vi "oa_TV Wait Until Ten Revs (NChan).vi"(5 "reset? (F)":bool, 8 "error in (no error)":errorcluster, 10 "pulse/revolution":i32[](array[numeric]), 11 "pulse position [s]":cluster{dbl[]}[](array[cluster]) {"?" format="%.2f"}) -> (0 "error out":errorcluster, 3 "pulse positions":cluster{dbl[]}[](array[cluster]))   [LabVIEW 2017, in "SoundVib_Torsional.lvlib"]
uses:
  <vilib>/addons/Sound and Vibration/Order Analysis/Torsional Vibration/SoundVib_Torsional.lvlib
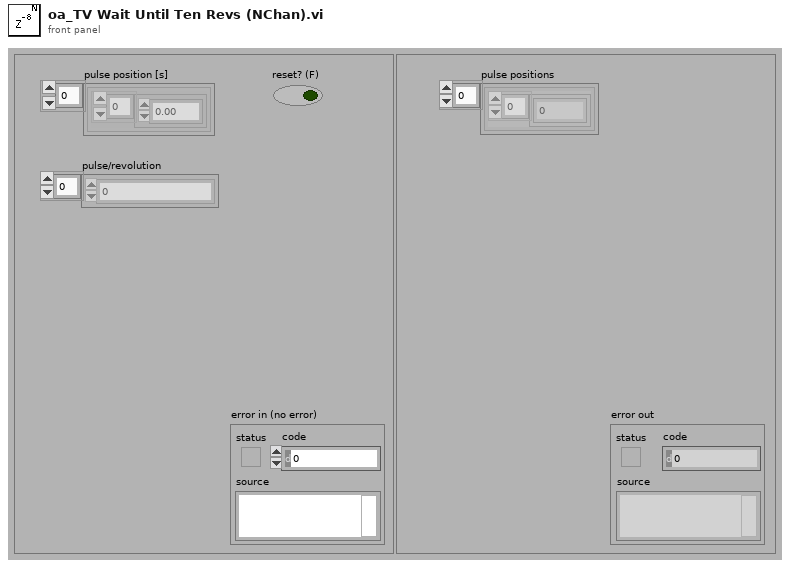
[diagram p1: front panel]
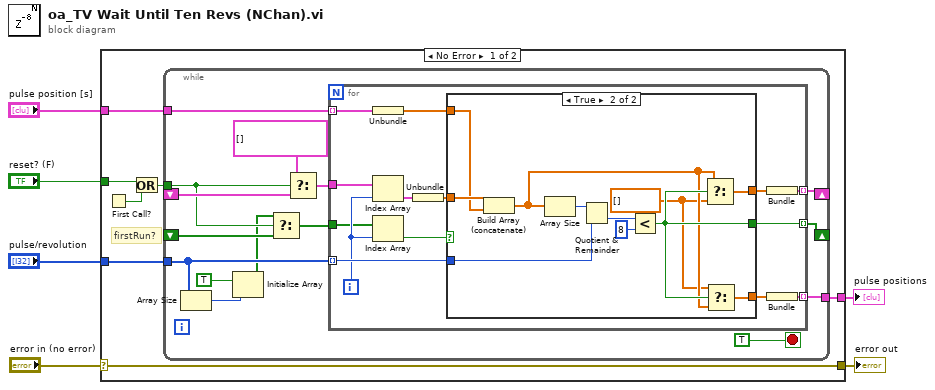
[diagram p0: block diagram]
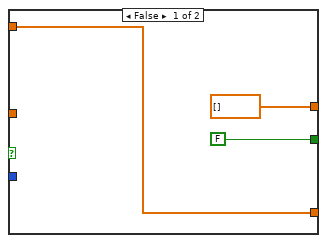
[diagram p2: hidden frame]
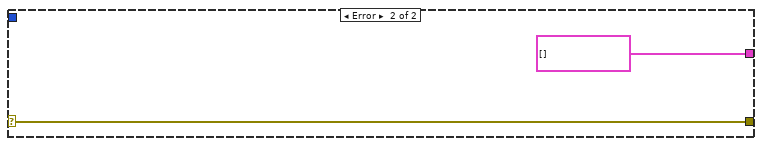
[diagram p3: hidden frame]
diagram:
  n1 = case shown="No Error" "error in (no error)" {
    selector: "error in (no error)" -> [w13 w58]
    tunnel: [w13 w58] -> w5
    tunnel: [w12 cluster{"f":dbl[]}[] []] -> w1
    tunnel: "reset? (F)" -> [w10 _]
    tunnel: "pulse position [s]" -> [w8 _]
    tunnel: "pulse/revolution" -> [w7 _]
    frame No Error {
      # "firstRun?"
      n2 = First Call?() -> (First Call?: T/F=w11:bool)
      n3 = Or(x=w10, y=w11) -> (x .or. y?=w9:bool)
      n4 = while {
        shift-right: [w24] -> _
        shift-left: _ -> [w23]
        tunnel: w9 -> [w19]
        shift-right: [w26] -> _
        shift-left: _ -> [w21]
        tunnel: [w25] -> w12
        tunnel: w8 -> [w20]
        tunnel: w7 -> [w18]
        stop <- TRUE stop-if-true
        n5 = Array Size(array=w18) -> (size(s)=w15:i32)
        n6 = Initialize Array(TRUE, w15) -> (w14:bool[])
        n7 = Select(t=w14, s=w19, f=w21) -> (s? t:f=w27:bool[])
        n8 = Select(t=cluster{dbl[]}[] [] ("pulse position [s]"), s=w19, f=w23) -> (s? t:f=w22:cluster{"f":dbl[]}[])
        n9 = for {
          tunnel: [w38] -> w25 mode=indexing
          tunnel: w20 -> [w42] mode=indexing
          tunnel: w18 -> [w40] mode=indexing
          tunnel: w22 -> [w37]
          tunnel: [w30] -> w24 mode=indexing
          tunnel: w27 -> [w31]
          tunnel: [w29] -> w26 mode=indexing
          i -> [w32]
          n10 = Unbundle(w42) -> (w41:dbl[])
          n11 = Index Array(array=w37, index=w32) -> (element=w36:cluster{"f":dbl[]})
          n12 = Index Array(array=w31, index=w32) -> (element=w33:bool)
          n13 = Unbundle(w36) -> ("f"=w35:dbl[])
          n14 = case shown="True" w33 {
            tunnel: [FALSE w55] -> w29
            tunnel: [w43 w53] -> w39
            tunnel: w40 -> [_ w51]
            tunnel: w35 -> [_ w49]
            tunnel: w41 -> [w43 w48]
            tunnel: [dbl[] [] ("pulse positions(2D)") w47] -> w34
            frame False {
            }
            frame True {
              w46 = dbl[] [] ("f")
              n15 = Build Array (concatenate)(w49, w48) -> (w54:dbl[])
              n16 = Array Size(array=w54) -> (size(s)=w52:i32)
              n17 = Quotient & Remainder(x=w52, y=w51) -> (floor(x/y)=w50:i32)  [unwired: 1 out]
              n18 = Less?(x=w50, y=8) -> (x < y?=w55:bool)
              n19 = Select(t=w54, s=w55, f=w46) -> (s? t:f=w47:dbl[])
              n20 = Select(t=w46, s=w55, f=w54) -> (s? t:f=w53:dbl[])
            }
          }
          n21 = Bundle("f"=w34) -> (w30:cluster{"f":dbl[]})  [unwired: 1 in]
          n22 = Bundle("f"=w39) -> (w38:cluster{"f":dbl[]})  [unwired: 1 in]
        }
      }
    }
    frame Error {
    }
  }
  "error out" <- w5
  "pulse positions" <- w1
